vi "Initialize.vi"(6 "Write delay (ms)":u32=1000, 7 "buffer size":i32=4096, 8 "error in (no error)":errorcluster, 10 "Enable? (T)":bool=TRUE, 11 "File path":path) -> (0 "error out":errorcluster, 3 "Logger out":refnum<class "Logger.lvclass">)   [LabVIEW 2011, in "Logger.lvclass"]
doc: "This VI returns an instance of the Logger class., which can be used to reference it again later on in the program. It also starts the logger itself, allowing data to be written in the background.\n\nEVERY initialize logger must have a corresponding close logger! Otherwise the logger will continue to run in the background."
uses:
  Logger.lvclass
  Logger.lvclass/Logger.ctl
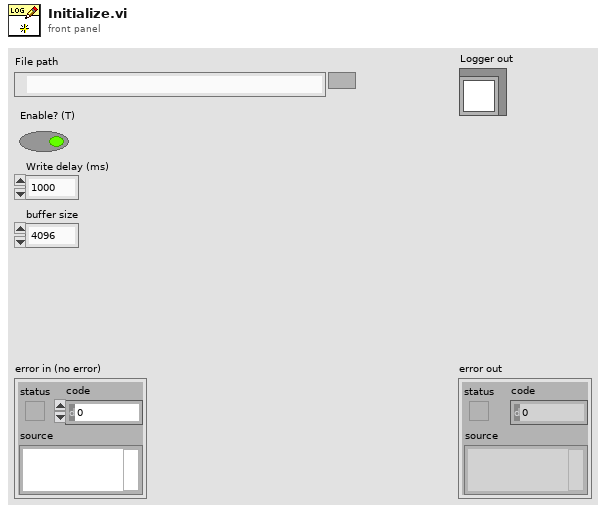
[diagram p1: front panel]
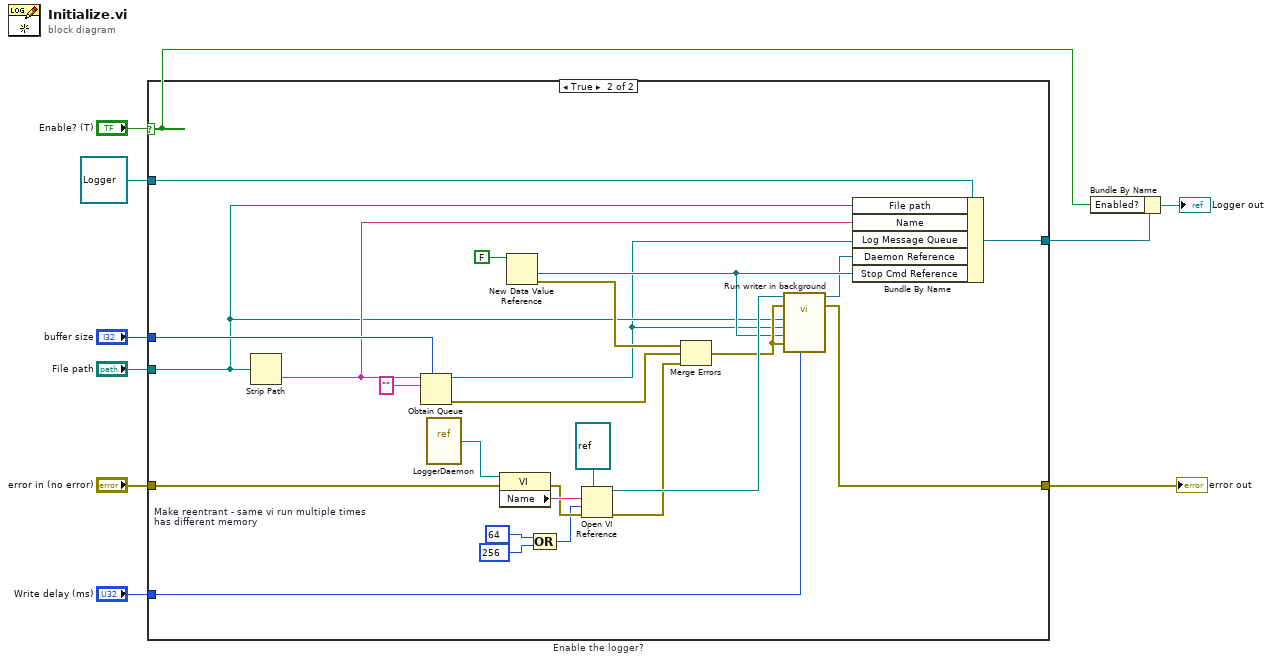
[diagram p0: block diagram]
diagram:
  n1 = case "Enable the logger?" shown="True" "Enable? (T)" {
    tunnel: "buffer size" -> [_ w36]
    tunnel: [w10 w20] -> w8
    tunnel: "error in (no error)" -> [w10 w18]
    tunnel: [w11 w17] -> w3
    tunnel: "Write delay (ms)" -> [_ w16]
    tunnel: "File path" -> [_ w15]
    tunnel: refnum<class "Logger.lvclass"> refnum ("NetworkStreamWriter in") -> [w11 w12]
    frame False {
    }
    frame True {
      w26 = 64  # Make reentrant - same vi run multiple times has different memory
      n2 = Strip Path(path=w15) -> (name=w19:string)  [unwired: 1 out]
      n3 = Obtain Queue(max queue size (-1, unlimited)=w36, name (unnamed)=w19, element data type="" ("name (unnamed)")) -> (queue out=w14:refnum<queue>, error out=w29:errorcluster)  [unwired: 2 in, 1 out]
      n4 = vi-ref "LoggerDaemon.vi"() -> (w35:refnum<vi>)
      n5 = property class="VI"(reference=w35, error in=w18) -> (error out=w31:errorcluster, "Name"=w34:string)  [unwired: 1 out]
      n6 = New Data Value Reference(data value=FALSE) -> (data value reference=w22:refnum<data-value>, error out=w23:errorcluster)  [unwired: 1 in]
      n7 = Compound Arithmetic op=OR(w26, 256 ("options")) -> (w25:i32)
      n8 = Open VI Reference(type specifier VI Refnum (for type only)=refnum<vi> refnum, vi path=w34, options=w25, error in (no error)=w31) -> (vi reference=w33:refnum<vi>, error out=w30:errorcluster)  [unwired: 2 in]
      n9 = Merge Errors(w23, w29, w30) -> (w28:errorcluster)
      n10 = call-by-ref "Run writer in background"(reference=w33, error in=w28, "Write delay (ms)"=w16, 8:"error in (no error)"=w28, "Stop Cmd Reference"=w22, "Log Message Queue"=w14, "File path"=w15) -> (reference out=w13:refnum<vi>, error out=w20:errorcluster)  [unwired: 6 in, 1 out]
      n11 = Bundle By Name(cluster=w12, "File path"=w15, "Name"=w19, "Log Message Queue"=w14, "Daemon Reference"=w13, "Stop Cmd Reference"=w22) -> (w17:refnum<class "Logger.lvclass">)
    }
  }
  "error out" <- w8
  n12 = Bundle By Name(cluster=w3, "Enabled?"="Enable? (T)") -> (→"Logger out":refnum<class "Logger.lvclass">)
